vi "CalculateSpecificationBuildOrder.vi"(6 "UpdateList":T1, 8 "error in (no error)":errorcluster, 11 "SolutionBuilder in":refnum<class "SolutionBuilder.lvclass">) -> (0 "error out":errorcluster, 3 "SolutionBuilder out":refnum<class "SolutionBuilder.lvclass">)   [LabVIEW 2019, in "SolutionBuilder.lvlib" / "SolutionBuilder.lvclass"]
uses:
  SolutionBuilder.lvclass
  Events/EventUpdateList.ctl
  SolutionBuilder.lvclass/SolutionBuilder.ctl
  SolutionBuilder.lvlib
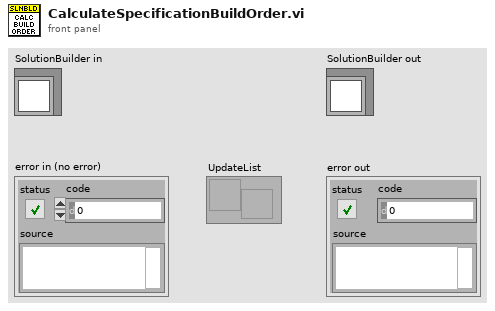
[diagram p1: front panel]
types:
  T1 = typedef "SolutionBuilder.lvlib/EventUpdateList.ctl" = refnum<user-event>
  T2 = typedef "SolutionBuilder.lvlib/SolutionBuilder.lvclass/OrderingMap.ctl" = map{cluster{"Owning project":path, "Build spec name":string, "Target":string}, cluster{"ProjectItem out":refnum<class "ProjectItem.lvclass">, "Deps":set{string}}}
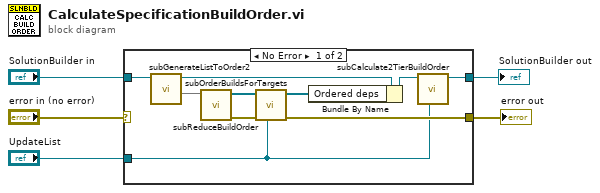
[diagram p0: block diagram]
diagram:
  n1 = case shown="No Error" "error in (no error)" {
    selector: "error in (no error)" -> [_ w17]
    tunnel: "UpdateList" -> [w6 _]
    tunnel: "SolutionBuilder in" -> [w15 w16]
    tunnel: [w12 w16] -> w3
    tunnel: [w7 w17] -> w1
    frame No Error {
      n2 = call "subGenerateListToOrder2.vi"("SolutionBuilder in"=w15) -> ("Ordering map"=w11:T2, "SolutionBuilder out"=w14:refnum<class "SolutionBuilder.lvclass">)  [unwired: 8 in, 1 out]
      n3 = call "subReduceBuildOrder.vi"("Ordering map"=w11) -> ("error out"=w8:errorcluster, "Raw build order"=w10:refnum<class "ProjectItem.lvclass">[])  [unwired: 9 in]
      n4 = call "subOrderBuildsForTargets.vi"("User Event in"=w6, "error in"=w8, "Raw build order in"=w10) -> ("error out"=w7:errorcluster, "Build order"=w9:refnum<class "ProjectItem.lvclass">[])  [unwired: 7 in]
      n5 = Bundle By Name(cluster=w14, "Ordered deps"=w9) -> (w13:refnum<class "SolutionBuilder.lvclass">)
      n6 = call "subCalculate2TierBuildOrder.vi"("UpdateList"=w6, "SolutionBuilder in"=w13) -> ("SolutionBuilder out"=w12:refnum<class "SolutionBuilder.lvclass">)  [unwired: 8 in, 1 out]
    }
    frame Error {
    }
  }
  "error out" <- w1
  "SolutionBuilder out" <- w3
